vi "Setup and Force DCPower Zero Voltage.vi"(7 "Channel Groups?":bool, 8 "error in":errorcluster, 9 "Parameters":T1={"Supply"=0.0, "Limit"=0.0, "Aperture Time"=0.0, "Settling Time"=0.0, "Sense"=1008, "Transient Response"=1041} {"Transient Response" items=["Slow"=1041, "Normal"=1038, "Fast"=1039, "Custom"=1042]; "Sense" items=["Local"=1008, "Remote"=1009]}, 10 "Channel List":string, 11 "DCPower Handle In":refnum<k15>) -> (0 "error out":errorcluster, 3 "DCPower Handle Out":refnum<k15>)   [LabVIEW 2021, in "PMIC Common.lvlib"]
uses:
  PMIC Common.lvlib
  DCPower Parameters.ctl
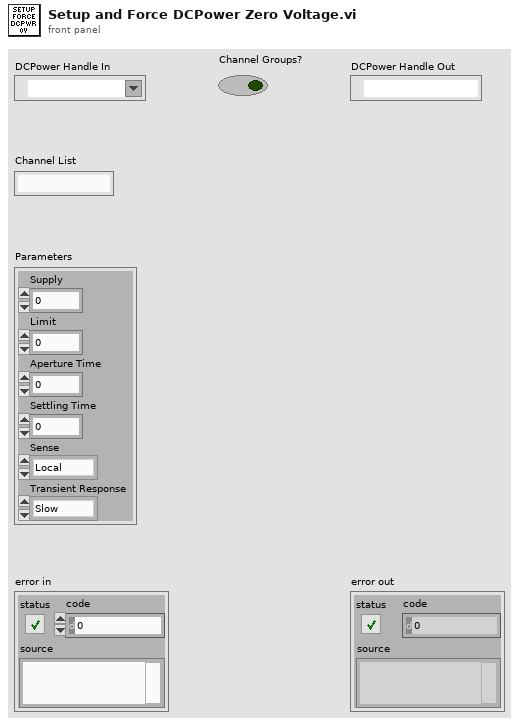
[diagram p1: front panel]
types:
  T1 = typedef "PMIC Common.lvlib/DCPower Parameters.ctl" = cluster{"Supply":dbl, "Limit":dbl, "Aperture Time":dbl, "Settling Time":dbl, "Sense":i32, "Transient Response":i32}
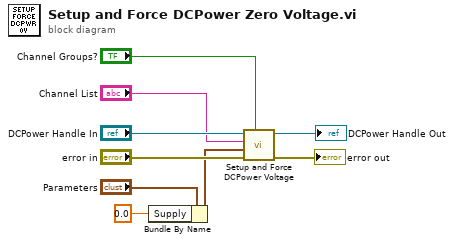
[diagram p0: block diagram]
diagram:
  n1 = Bundle By Name(cluster="Parameters", "Supply"=0.0) -> (w5:T1)
  n2 = call "Setup and Force DCPower Voltage.vi"("Channel Groups?"="Channel Groups?", "error in"="error in", "Parameters"=w5, "Channel List"="Channel List", "DCPower Handle In"="DCPower Handle In") -> ("error out"=→"error out":errorcluster, "DCPower Handle Out"=→"DCPower Handle Out":refnum<k15>)  [unwired: 5 in]
